vi "Dispense.vi"(8 "error in (no error)":errorcluster, 11 "Ultimus V in":refnum<class "Ultimus V.lvclass">) -> (0 "error out":errorcluster, 3 "Ultimus V out":refnum<class "Ultimus V.lvclass">)   [LabVIEW 2020, in "Ultimus V.lvclass"]
uses:
  Ultimus V.lvclass
  Ultimus V.lvclass/Ultimus V.ctl
  EFD Ultimus V/EFD Ultimus V.lvlib
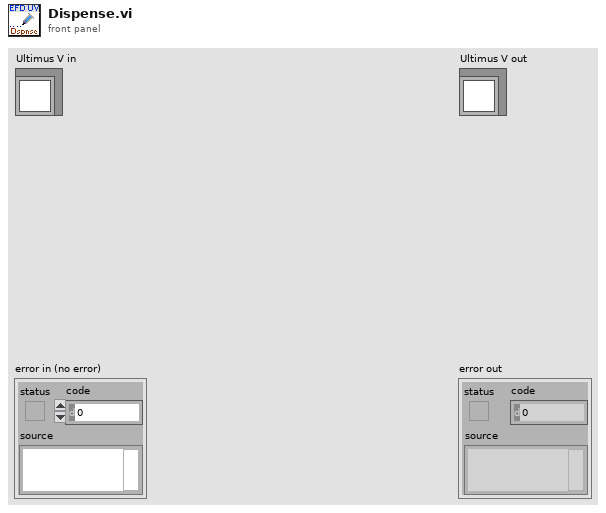
[diagram p1: front panel]
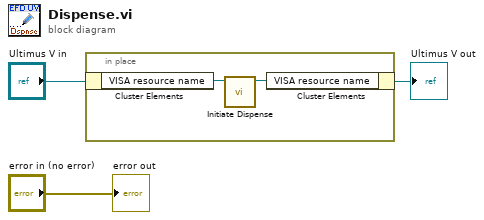
[diagram p0: block diagram]
diagram:
  n1 = in-place {
    n2 = in-place-cluster #1("Ultimus V in") -> ("VISA resource name"=w4:refnum<visa-resource-name>)
    n3 = call "Initiate Dispense.vi"("VISA resource name"=w4) -> ("VISA resource name out"=w5:refnum<visa-resource-name>)  [unwired: 9 in, 1 out]
    n4 = in-place-cluster #1("VISA resource name"=w5) -> (→"Ultimus V out":refnum<class "Ultimus V.lvclass">)
  }
  "error out" <- "error in (no error)"
